vi "Created Aliases.vi"(11 "jettl Actor in":refnum<class "jettl Actor.lvclass">) -> (2 "Created Aliases":T1)   [LabVIEW 2021, in "jettl.lvlib" / "Temporary Actor.lvlib" / "jettl Actor.lvclass"]
uses:
  jettl Actor.lvclass
  Utilities/Created Aliases.ctl
  jettl Actor.lvclass/jettl Actor.ctl
  Addresses Strategy/Addresses Strategy/Addresses Strategy.lvclass
  Utilities/Utilities.lvlib
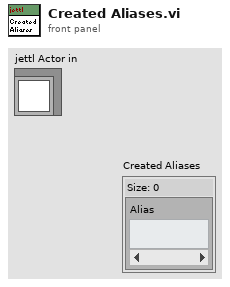
[diagram p1: front panel]
types:
  T1 = typedef "jettl.lvlib/Utilities.lvlib/Created Aliases.ctl" = set{string}
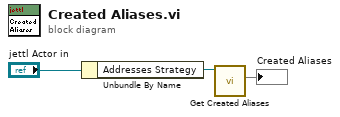
[diagram p0: block diagram]
diagram:
  n1 = Unbundle By Name("jettl Actor in") -> ("Addresses Strategy"=w3:refnum<class "Addresses Strategy.lvclass">)
  n2 = call-dynamic "Get Created Aliases.vi"("Addresses Strategy in"=w3) -> ("Created Aliases"=→"Created Aliases":T1)  [unwired: 10 in]
